vi "Measurement UI.vi"() -> ()   [LabVIEW 2025, in "CAN-LIN Raw Bus Capture UI.lvlib"]
uses:
  CAN-LIN Raw Bus Capture UI.lvlib
  Toggle.ctl
  <vilib>/Utility/file.llb/Write Delimited Spreadsheet (string).vi
  Table_Filtering/Table_Filtering.lvlib
panel:
  in  "STOP":bool
  out "last  update":u32
  out "Connection":bool
  in  "Clear Trace":bool
  in  "Captured Data":string[][](array[string])
  in  "Bus Type":string
  in  "Lin Interface":string
  out "Message Buffer":string[][](table)
  in  "Can Interface":string
  in  "Path":path
  in  "Save to CSV":bool
  in  "Filter":string
  in  "SortByID":bool
  out "Status":string
  out "Trace":string[][](table)
  in  "SETTINGS":enum32{"CAN", "LIN"}(tab)
  in  "DUT Pin":string(combo) caption="Pin name"
  in  "IO Mode":enum32{"CAN", "CAN FD", "CAN FD + BRS"}(ring)
  in  "FD ISO Mode":enum32{"ISO", "Non ISO", "Legacy ISO"}(ring)
  in  "Baudrate":u32 format="%x"
  in  "FD Baudrate":u32 format="%x"
  in  "Termination CAN":T1
  in  "INTERFACE NAME CAN":refnum<k21>
  in  "Timeout (s)":u32
  in  "Termination LIN":T1
  in  "INTERFACE NAME LIN":refnum<k21>
  # "CONFIGURATION"
  # "CONTROL"
  # "TRACE"
  # "STATUS"
  # "CAN Settings"
  # "LIN Settings"
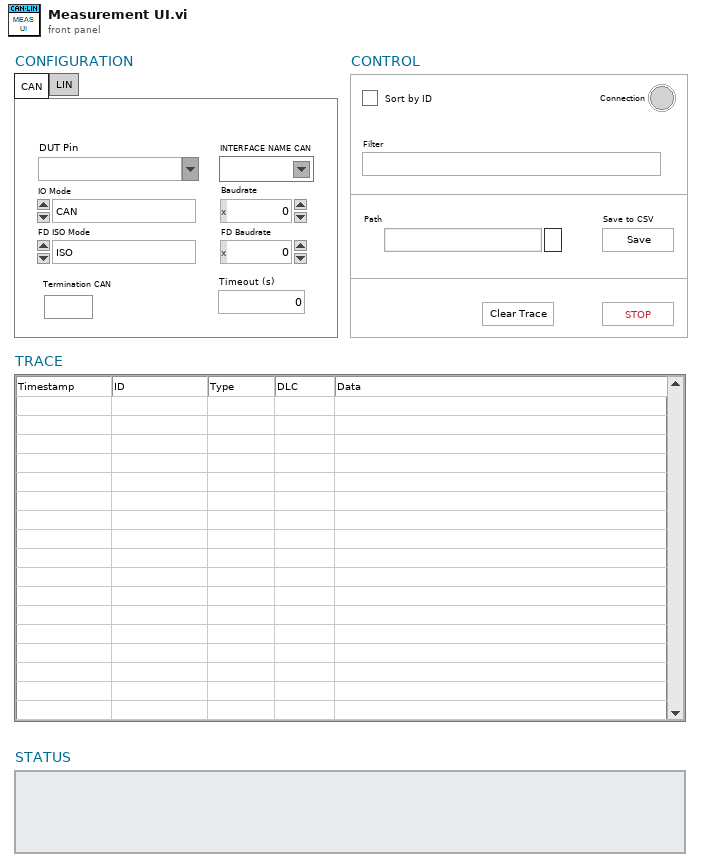
[diagram p1: front panel]
types:
  T1 = typedef "Toggle.ctl" = bool
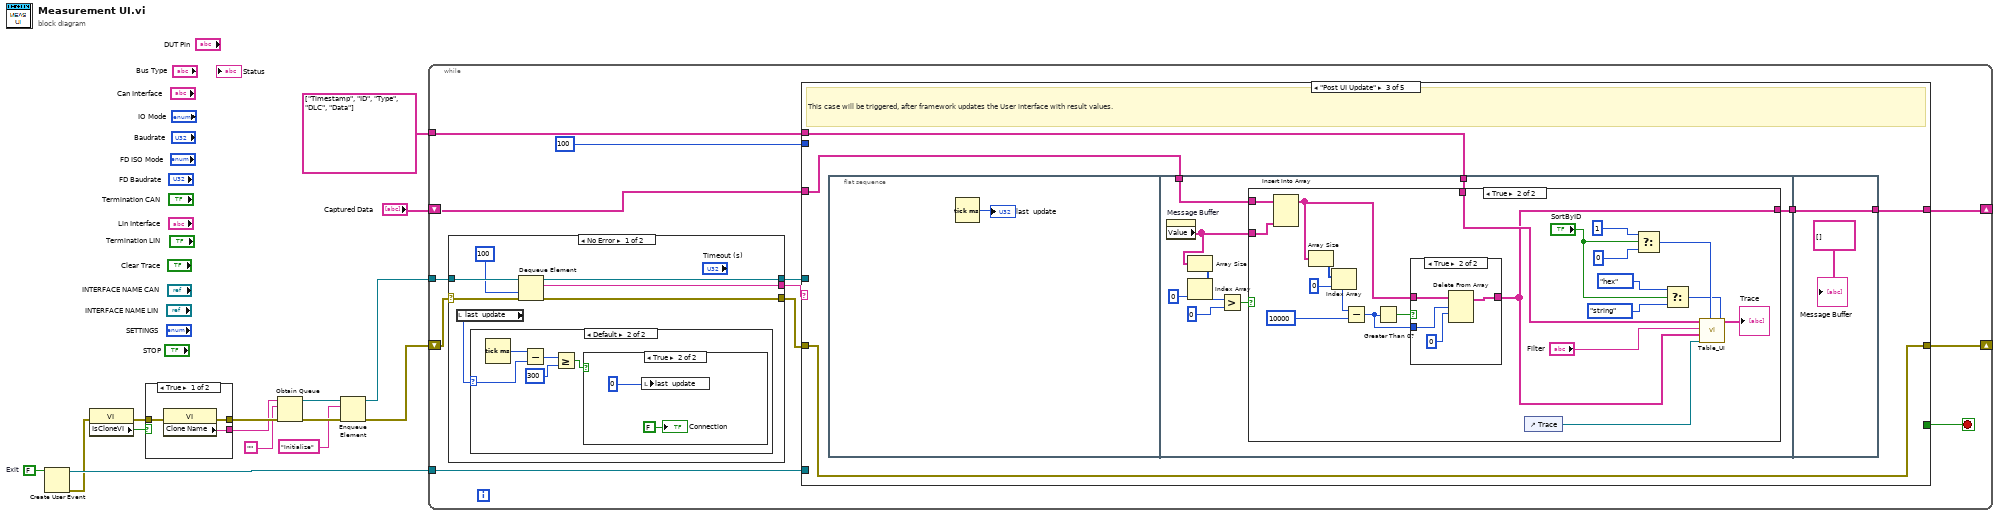
[diagram p0: block diagram]
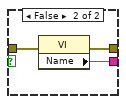
[diagram p2: hidden frame]
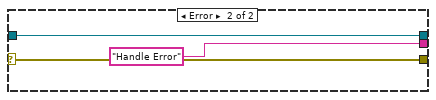
[diagram p5: hidden frame]
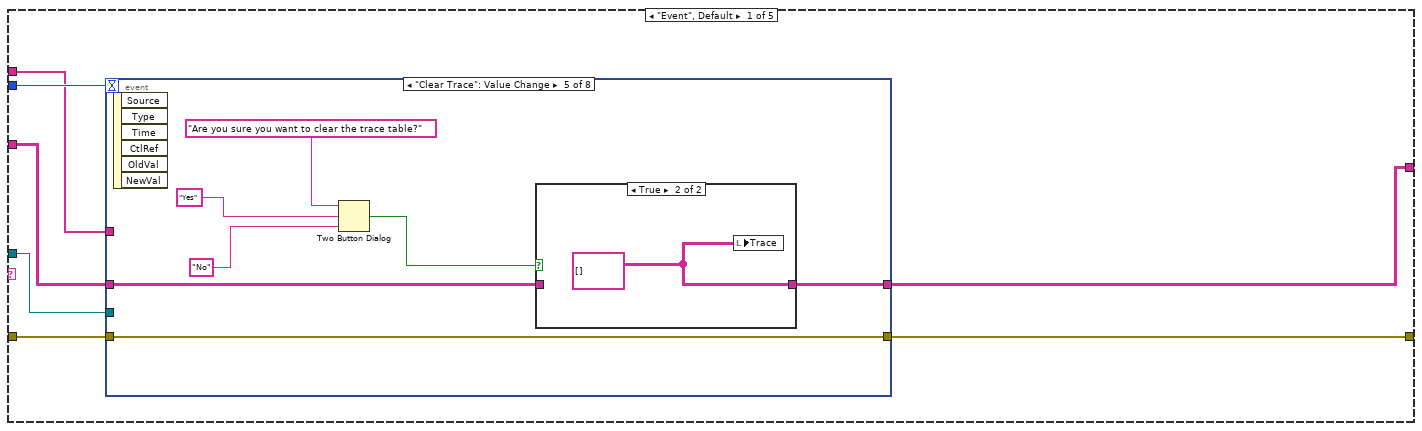
[diagram p6: hidden frame]
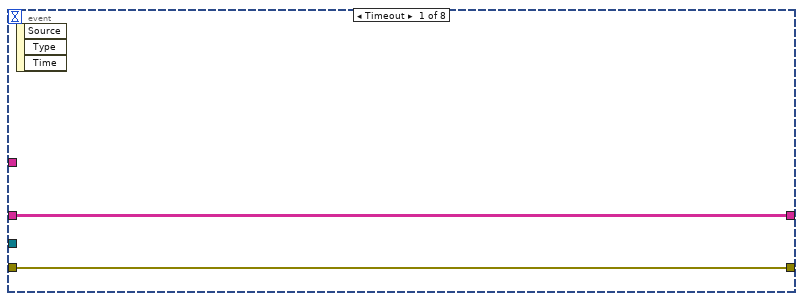
[diagram p7: hidden frame]
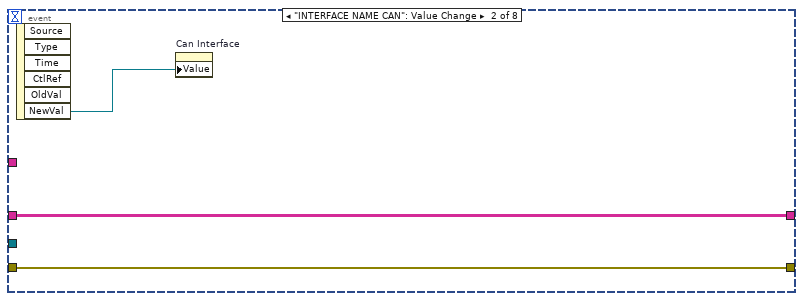
[diagram p8: hidden frame]
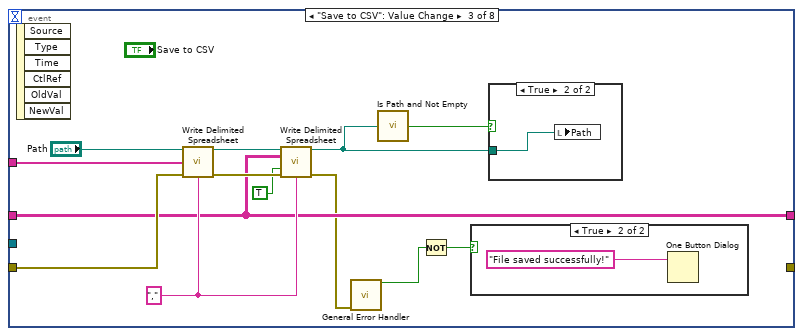
[diagram p9: hidden frame]
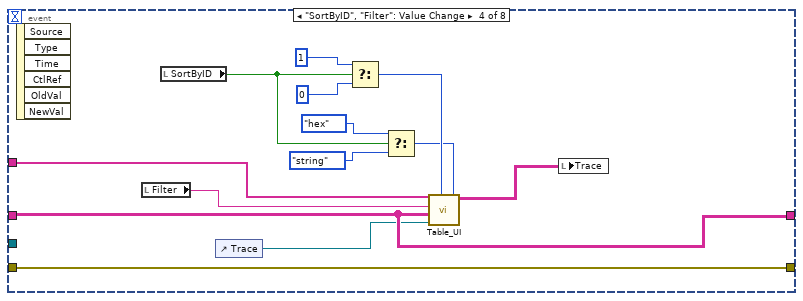
[diagram p12: hidden frame]
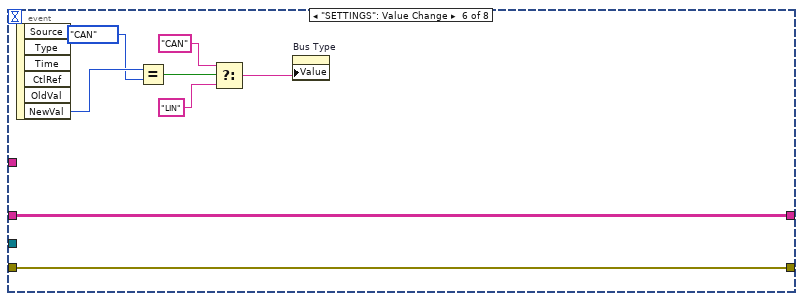
[diagram p14: hidden frame]
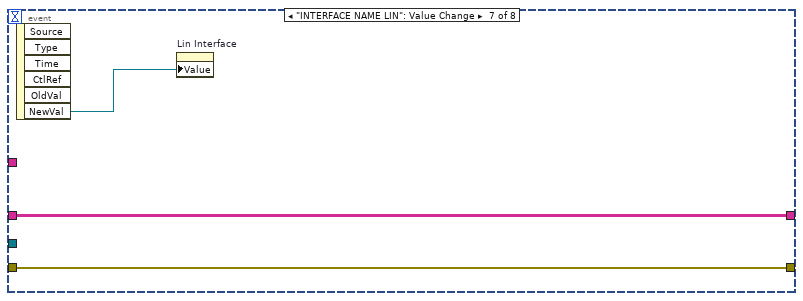
[diagram p15: hidden frame]
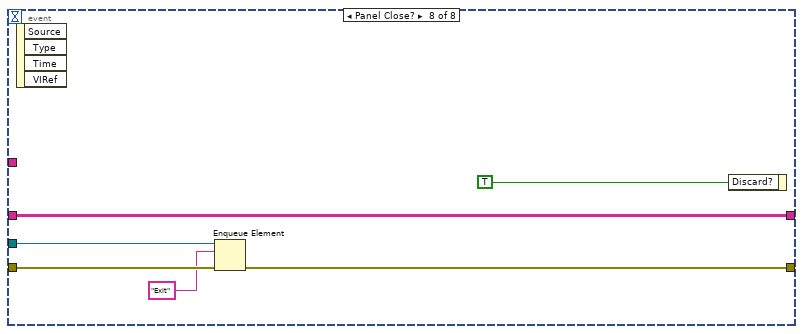
[diagram p16: hidden frame]
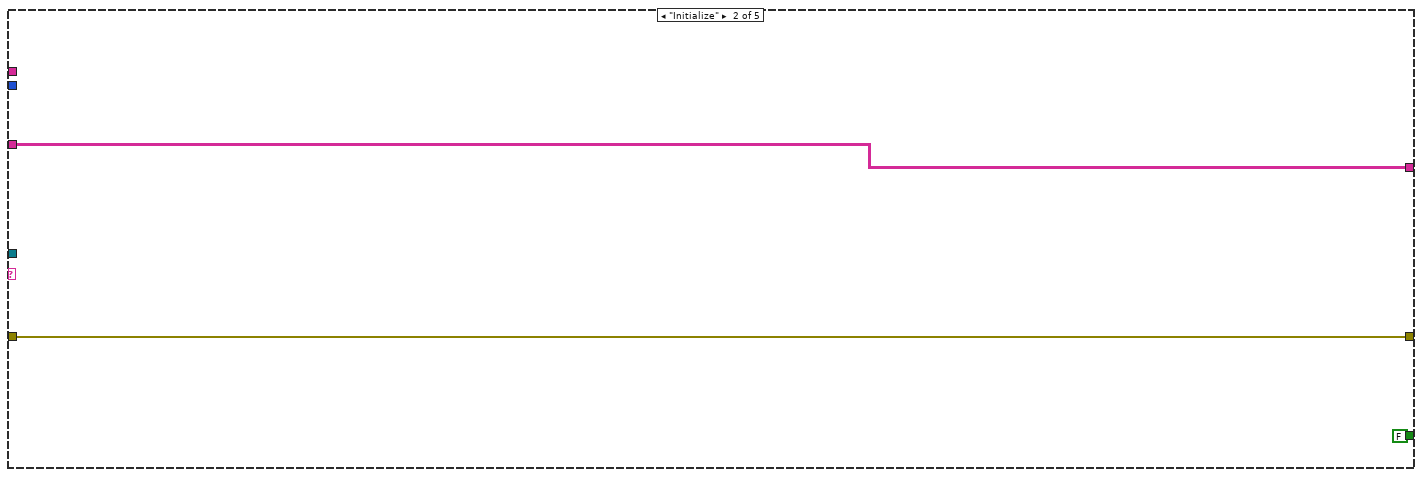
[diagram p17: hidden frame]
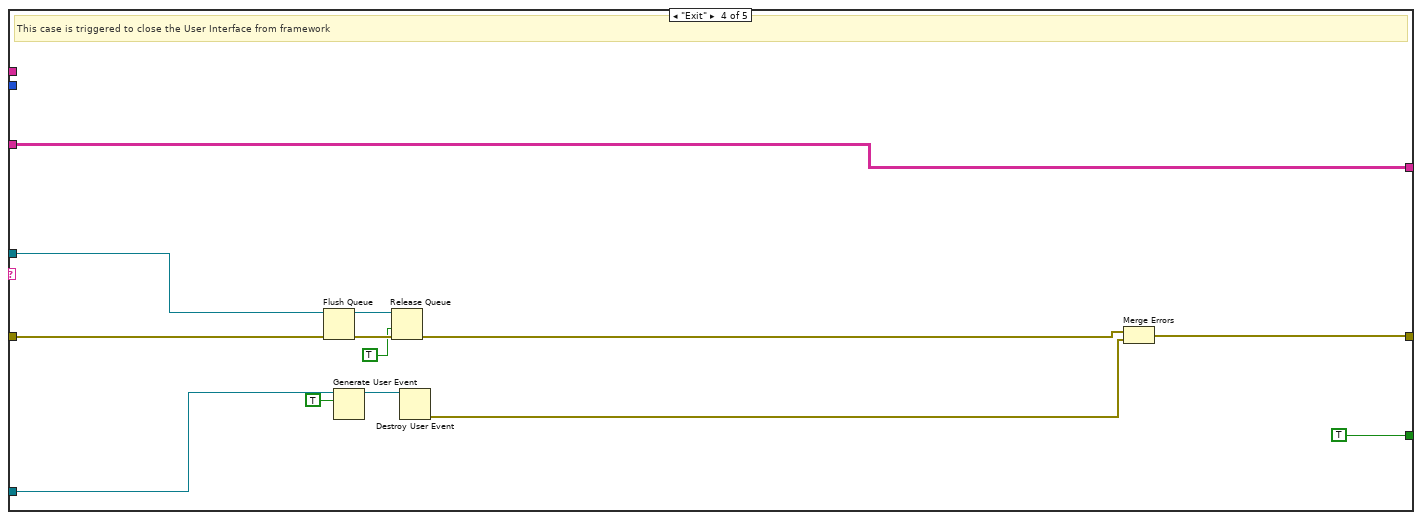
[diagram p20: hidden frame]
diagram:
  w5 = FALSE  # Exit
  n1 = Create User Event(user event datatype=w5) -> (user event=w4:refnum<user-event>, error out=w3:errorcluster)  [unwired: 1 in]
  n2 = property class="VI"(error in=w3) -> (error out=w6:errorcluster, "IsCloneVI"=w7:bool)  [unwired: 1 in, 1 out]
  n3 = case shown="True" w7 {
    tunnel: [w18 w21] -> w15
    tunnel: [w17 w20] -> w14
    tunnel: w6 -> [w16 w19]
    frame True {
      n4 = property class="VI"(error in=w16) -> (error out=w18:errorcluster, "Clone Name"=w17:string)  [unwired: 1 in, 1 out]
    }
    frame False {
      n5 = property class="VI"(error in=w19) -> (error out=w21:errorcluster, "Name"=w20:string)  [unwired: 1 in, 1 out]
    }
  }
  n6 = Obtain Queue(name (unnamed)=w14, element data type="", error in (no error)=w15) -> (queue out=w11:refnum<queue>, error out=w13:errorcluster)  [unwired: 2 in, 1 out]
  n7 = Enqueue Element(queue=w11, element="Initialize", error in (no error)=w13) -> (queue out=w10:refnum<queue>, error out=w12:errorcluster)  [unwired: 1 in, 1 out]
  n8 = while {
    shift-right: [w28] -> _
    shift-left: w12 -> [w33]
    tunnel: w10 -> [w31]
    tunnel: w4 -> [w26]
    tunnel: string[] ["Timestamp", "ID", "Type", "DLC", "Data"] ("Headers") -> [w24]
    shift-right: [w22] -> _
    shift-left: "Captured Data" -> [w23]
    stop <- w27 stop-if-true
    n9 = case shown="No Error" w33 {
      selector: w33 -> [w40 w50]
      tunnel: [w39 w50] -> w32
      tunnel: w31 -> [w38 w49]
      tunnel: [w37 w49] -> w30
      tunnel: [w36 "Handle Error"] -> w29
      frame No Error {
        n10 = local read "last  update"() -> (w34:u32)
        n11 = case shown="Default" w34 {
          selector: w34 -> [_ w44]
          frame 0 {
          }
          frame Default {
            n12 = Tick Count (ms)() -> (millisecond timer value=w45:u32)
            n13 = Subtract(x=w45, y=w44) -> (x-y=w43:u32)
            n14 = Greater Or Equal?(x=w43, y=u32 300) -> (x >= y?=w41:bool)
            n15 = case shown="True" w41 {
              frame False {
              }
              frame True {
                n16 = local write "last  update"(u32 0 ("last  update")) -> ()
                "Connection" <- FALSE ("Connection")
              }
            }
          }
        }
        n17 = Dequeue Element(queue=w38, timeout in ms (-1)=100, error in (no error)=w40) -> (queue out=w37:refnum<queue>, element=w36:string, error out=w39:errorcluster)  [unwired: 1 out]
      }
      frame Error {
      }
    }
    n18 = case shown="\"Post UI Update\"" w29 {
      tunnel: w32 -> [w56 w119 w124 w176 w179]
      tunnel: w30 -> [w55 _ _ w174 w178]
      tunnel: [w57 w119 w124 w167 w179] -> w28
      tunnel: [_ FALSE _ TRUE _] -> w27
      tunnel: w26 -> [_ _ _ w168 _]
      tunnel: 100 -> [w54 _ _ _ _]
      tunnel: w24 -> [w53 _ w123 _ _]
      tunnel: w23 -> [w51 w117 w122 w164 w177]
      tunnel: [w52 w117 w121 w164 w177] -> w22
      frame "Event", Default {
        n19 = event shown="[4] \"Clear Trace\": Value Change" {
          selector: _ -> [_ _ _ _ _ _ _ _]
          dyn-events: _ -> [_ _ _ _ _ _ _ _]
          timeout: w54 -> [_ _ _ _ _ _ _ _]
          tunnel: [w59 w61 _ w84 w91 w101 w109 w114] -> w57
          tunnel: w56 -> [w59 w61 w74 w84 w91 w101 w109 w115]
          tunnel: w55 -> [_ _ _ _ _ _ _ w113]
          tunnel: w51 -> [w58 w60 w66 w80 w92 w100 w108 w111]
          tunnel: w53 -> [_ _ w71 w81 _ _ _ _]
          tunnel: [w58 w60 w66 w80 w97 w100 w108 w111] -> w52
          event Timeout {
            n20 = event-data() -> ()  [unwired: 1 in, 3 out]
          }
          event "INTERFACE NAME CAN": Value Change {
            n21 = event-data() -> ("NewVal"=w62:refnum<k21>)  [unwired: 1 in, 5 out]
            n22 = property on="Can Interface" class="Str"("Value"=w62) -> ()  [unwired: 2 in, 2 out]
          }
          event "Save to CSV": Value Change {
            w69 = "," ("delimiter (\\t)")
            n23 = event-data() -> ()  [unwired: 1 in, 6 out]
            n24 = call-poly <vilib>:"Write Delimited Spreadsheet.vi"("file path (dialog if empty)"="Path", "1D data"=w71, "error in (no error)"=w74, "delimiter (\\t)"=w69) -> ("new file path (Not A Path if cancelled)"=w70:path, "error out"=w73:errorcluster)  [unwired: 10 in]
            n25 = call-poly <vilib>:"Write Delimited Spreadsheet.vi"("file path (dialog if empty)"=w70, "2D data"=w66, "append to file? (new file:F)"=TRUE, "error in (no error)"=w73, "delimiter (\\t)"=w69) -> ("new file path (Not A Path if cancelled)"=w67:path, "error out"=w65:errorcluster)  [unwired: 9 in]
            n26 = call <vilib>:"General Error Handler.vi"("error in (no error)"=w65) -> ("error?"=w63:bool)  [unwired: 10 in, 4 out]
            n27 = call <vilib>:"Is Path and Not Empty.vi"("path"=w67) -> ("Is Path and Not Empty?"=w68:bool)  [unwired: 4 in]
            n28 = Not(x=w63) -> (.not. x?=w64:bool)
            n29 = case shown="True" w64 {
              frame False {
              }
              frame True {
                n30 = One Button Dialog(message="File saved successfully!") -> ()  [unwired: 1 in, 1 out]
              }
            }
            n31 = case shown="True" w68 {
              tunnel: w67 -> [_ w77]
              frame False {
              }
              frame True {
                n32 = local write "Path"(w77) -> ()
              }
            }
          }
          event "SortByID", "Filter": Value Change {
            n33 = event-data() -> ()  [unwired: 1 in, 6 out]
            n34 = local read "Filter"() -> (w82:string)
            n35 = local read "SortByID"() -> (w83:bool)
            n36 = control-ref of="Trace"() -> (w79:refnum<vi>)
            n37 = Select(t=1, s=w83, f=0) -> (s? t:f=w88:i32)
            n38 = Select(t=enum16{"numerical", "hex", "string"}."hex" ("Sort Type"), s=w83, f=enum16{"numerical", "hex", "string"}."string" ("Sort Type")) -> (s? t:f=w87:enum16{"numerical", "hex", "string"})
            n39 = call "Table_UI.vi"("Sort Type"=w87, "Sort by"=w88, "Table Control"=w79, "Prefiltered Data"=w80, "Filter String"=w82, "Headers"=w81) -> ("Table Control"=w78:string[][])  [unwired: 5 in]
            n40 = local write "Trace"(w78) -> ()
          }
          event "Clear Trace": Value Change {
            n41 = event-data() -> ()  [unwired: 1 in, 6 out]
            n42 = Two Button Dialog(message="Are you sure you want to clear the trace table?", 1:"No" ("F button name (\"Cancel\")"), 2:"Yes" ("T button name (\"OK\")")) -> (T button?=w93:bool)
            n43 = case shown="True" w93 {
              tunnel: [w98 w99] -> w97
              tunnel: w92 -> [w98 _]
              frame False {
              }
              frame True {
                w99 = string[][] [] ("Captured Data")
                n44 = local write "Trace"(w99) -> ()
              }
            }
          }
          event "SETTINGS": Value Change {
            n45 = event-data() -> ("NewVal"=w107:enum32{"CAN", "LIN"})  [unwired: 1 in, 5 out]
            n46 = Equal?(x=w107, y=enum32{"CAN", "LIN"}."CAN") -> (x = y?=w105:bool)
            n47 = Select(t="CAN", s=w105, f="LIN") -> (s? t:f=w102:string)
            n48 = property on="Bus Type" class="Str"("Value"=w102) -> ()  [unwired: 2 in, 2 out]
          }
          event "INTERFACE NAME LIN": Value Change {
            n49 = event-data() -> ("NewVal"=w110:refnum<k21>)  [unwired: 1 in, 5 out]
            n50 = property on="Lin Interface" class="Str"("Value"=w110) -> ()  [unwired: 2 in, 2 out]
          }
          event Panel Close? {
            n51 = event-data() -> ()  [unwired: 1 in, 4 out]
            n52 = Enqueue Element(queue=w113, element="Exit", error in (no error)=w115) -> (error out=w114:errorcluster)  [unwired: 1 in, 2 out]
            n53 = event-data("Discard?"=TRUE) -> ()  [unwired: 1 in, 1 out]
          }
        }
      }
      frame "Initialize" {
      }
      frame "Post UI Update" {
        # "This case will be triggered, after framework updates the User interface with result values."
        n54 = flat-sequence {
          tunnel: w123 -> [w132]
          tunnel: w122 -> [w134]
          tunnel: [w133] -> w120
          tunnel: [w162] -> w121
          tunnel: w120 -> [w162]
          frame #0 {
            n55 = Tick Count (ms)() -> (millisecond timer value=→"last  update":u32)
          }
          frame #1 {
            n56 = property on="Message Buffer" class="Tbl (strict)"() -> ("Value"=w131:string[][])  [unwired: 2 in, 2 out]
            n57 = Array Size(array=w131) -> (size(s)=w130:i32[])
            n58 = Index Array(array=w130, index=0) -> (element=w128:i32)
            n59 = Greater?(x=w128, y=0) -> (0:w126:bool)
            n60 = case shown="True" w126 {
              tunnel: w134 -> [w135 w154]
              tunnel: [w135 w136] -> w133
              tunnel: w132 -> [_ w151]
              tunnel: w131 -> [_ w144]
              frame False {
              }
              frame True {
                n61 = Insert Into Array(array=w154, new element=w144) -> (w137:string[][])  [unwired: 2 in]
                n62 = Array Size(array=w137) -> (size(s)=w143:i32[])
                n63 = Index Array(array=w143, index=0) -> (element=w141:i32)
                n64 = Subtract(x=w141, y=10000) -> (x-y=w138:i32)
                n65 = Greater Than 0?(x=w138) -> (x > 0?=w139:bool)
                n66 = case shown="True" w139 {
                  tunnel: w137 -> [w157 w161]
                  tunnel: w138 -> [_ w160]
                  tunnel: [w157 w158] -> w136
                  frame False {
                  }
                  frame True {
                    n67 = Delete From Array(array=w161, length=w160, index (row)=0) -> (array with subset deleted=w158:string[][])  [unwired: 1 in, 1 out]
                  }
                }
                n68 = control-ref of="Trace"() -> (w153:refnum<vi>)
                n69 = Select(t=1, s="SortByID", f=0) -> (s? t:f=w149:i32)
                n70 = Select(t=enum16{"numerical", "hex", "string"}."hex" ("Sort Type"), s="SortByID", f=enum16{"numerical", "hex", "string"}."string" ("Sort Type")) -> (s? t:f=w148:enum16{"numerical", "hex", "string"})
                n71 = call "Table_UI.vi"("Sort Type"=w148, "Sort by"=w149, "Table Control"=w153, "Prefiltered Data"=w136, "Filter String"="Filter", "Headers"=w151) -> ("Table Control"=→"Trace":string[][])  [unwired: 5 in]
              }
            }
          }
          frame #2 {
            "Message Buffer" <- string[][] [] ("Message Buffer")
          }
        }
      }
      frame "Exit" {
        # "This case is triggered to close the User Interface from framework"
        n72 = Flush Queue(queue=w174, error in (no error)=w176) -> (queue out=w173:refnum<queue>, error out=w172:errorcluster)  [unwired: 1 out]
        n73 = Generate User Event(user event=w168, event data cluster=TRUE ("event data")) -> (user event out=w170:refnum<user-event>)  [unwired: 2 in, 1 out]
        n74 = Release Queue(queue=w173, force destroy? (F)=TRUE, error in (no error)=w172) -> (error out=w166:errorcluster)  [unwired: 2 out]
        n75 = Destroy User Event(user event=w170) -> (error out=w165:errorcluster)  [unwired: 1 in]
        n76 = Merge Errors(w166, w165) -> (w167:errorcluster)
      }
      frame "Handle Error" {
        n77 = Unbundle By Name(w179) -> ("code"=w183:i32, "source"=w182:string)
        n78 = case shown="Default" w179 {
          selector: w179 -> [w184 w189]
          tunnel: [w184 w188] -> _
          tunnel: w178 -> [_ w185]
          frame No Error {
          }
          frame Default {
            n79 = call <vilib>:"Clear Errors.vi"("error in (no error)"=w189) -> ("error out"=w187:errorcluster)  [unwired: 5 in, 1 out]
            n80 = Enqueue Element At Opposite End(queue=w185, element="Exit", error in (no error)=w187) -> (error out=w188:errorcluster)  [unwired: 1 in, 2 out]
          }
        }
        n81 = Format Into String(initial string="UI main loop stopped, Error: " ("format string"), w183, "\r\n", w182) -> ()  [unwired: 2 in, 2 out]
      }
    }
  }
